vi "SampleMethod.vi"(8 "error in (no error)":errorcluster, 9 "Refnum in":refnum<k20>, 11 "SampleClass in":refnum<class "SampleClass.lvclass">) -> (0 "error out":errorcluster, 3 "SampleClass out":refnum<class "SampleClass.lvclass">)   [LabVIEW 2020, in "SampleLib.lvlib" / "SampleClass.lvclass"]
uses:
  SampleClass.lvclass
  ExternalClass/ExternalClass.lvclass
  SampleDependentClass/SampleDependentClass.lvclass
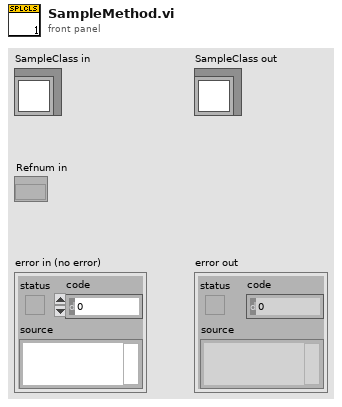
[diagram p1: front panel]
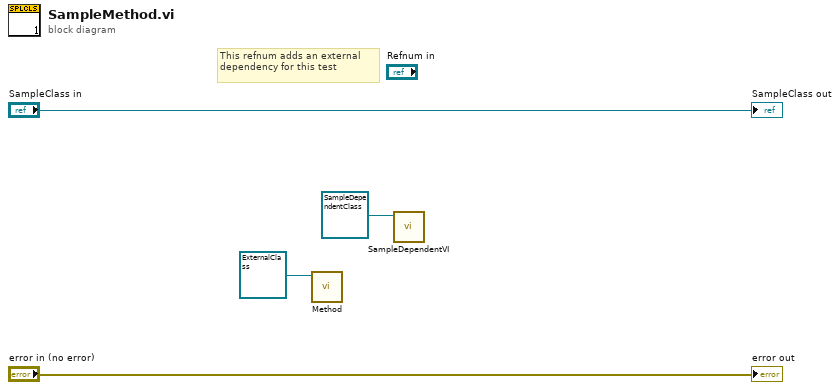
[diagram p0: block diagram]
diagram:
  # "This refnum adds an external dependency for this test"
  n1 = call-dynamic "Method.vi"("ExternalClass in"=refnum<class "ExternalClass.lvclass"> refnum) -> ()  [unwired: 9 in, 2 out]
  n2 = call-dynamic "SampleDependentVI.vi"("SampleDependentClass in"=refnum<class "SampleDependentClass.lvclass"> refnum) -> ()  [unwired: 9 in, 2 out]
  "error out" <- "error in (no error)"
  "SampleClass out" <- "SampleClass in"
